vi "logger.vi"(11 "error in (no error)":errorcluster) -> ()   [LabVIEW 2017, in "logger.lvlib"]
doc: "Log an error to a error.log file"
uses:
  logger.lvlib
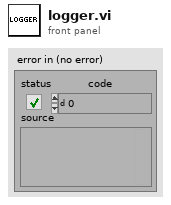
[diagram p1: front panel]
types:
  T1 = enum16{"open", "replace", "create", "open or create", "replace or create", "replace or create with confirmation"}
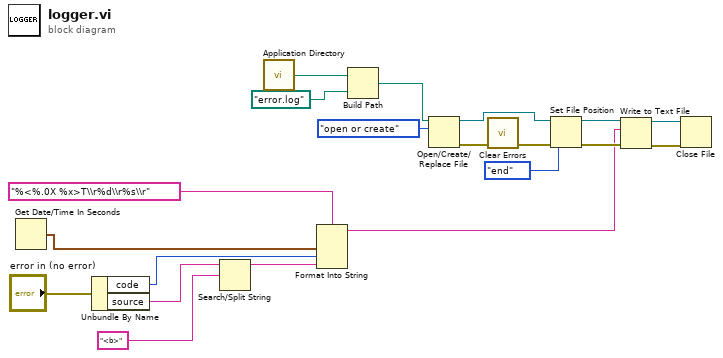
[diagram p0: block diagram]
diagram:
  n1 = Get Date/Time In Seconds() -> (seconds since 1Jan1904=w19:timestamp)
  n2 = Unbundle By Name("error in (no error)") -> ("code"=w18:i32, "source"=w16:string)
  n3 = Search/Split String(string=w16, search string/char (-)="<b>") -> (substring before match=w15:string)  [unwired: 1 in, 2 out]
  n4 = call <vilib>:"Application Directory.vi"() -> ("Application Directory"=w12:path)
  n5 = Format Into String(format string="%<%.0X %x>T\\r%d\\r%s\\r", w19, w18, w15) -> (resulting string=w3:string)  [unwired: 2 in, 1 out]
  n6 = Build Path(base path=w12, name or relative path=path "error.log") -> (appended path=w10:path)
  n7 = Open/Create/Replace File(file path (use dialog)=w10, operation (0:open)=T1."open or create") -> (refnum out=w7:refnum<file>, error out=w9:errorcluster)  [unwired: 4 in, 1 out]
  n8 = call <vilib>:"Clear Errors.vi"("error in (no error)"=w9) -> ("error out"=w8:errorcluster)  [unwired: 5 in, 1 out]
  n9 = Set File Position(refnum=w7, from (0:start)=enum16{"start", "end", "current"}."end", error in=w8) -> (refnum out=w4:refnum<file>, error out=w5:errorcluster)  [unwired: 1 in]
  n10 = Write to Text File(file (use dialog)=w4, text=w3, error in=w5) -> (refnum out=w1:refnum<file>, error out=w2:errorcluster)  [unwired: 1 in, 1 out]
  n11 = Close File(refnum=w1, error in=w2) -> ()  [unwired: 2 out]
